vi "fucking cubes.vi"() -> ()   [LabVIEW 2010]
uses:
  <vilib>/Analysis/Matrix/Datatypes/RealMatrix.ctl
  <vilib>/picture/3D Picture Control/NI_3D Picture Control.lvlib
  <vilib>/Analysis/Matrix/NI_Matrix.lvlib
panel:
  out "Supercell Structure":T1={"Structure Name"="A3B3_twin", "Lattice vector a"=[4.67354, 0.0, 0.0], "Lattice vector b"=[0.0, 8.0948, 0.0], "Lattice vector c"=[0.0, 0.0, 22.8956], "Atoms Array"=[{"Atom Name"="Cd", "Positions (Direct)"=[[0.0, 0.3333160110632741, 0.0416917449166463], [0.5000009999999975, 0.8333170110632716, 0.0416917449166463], [0.5000009999999975, 0.1666621408709168, 0.208337818520255], [0.0, 0.6666631408709214, 0.208337818520255], [0.0, 8.4662249422e-06, 0.3749383421346864], [0.5000009999999975, 0.5000094662249397, 0.3749383421346864], [0.0, -8.4662249422e-06, 0.8749383421346864], [0.5000009999999975, 0.4999925337750553, 0.8749383421346864], [0.0, 0.3333388591290807, 0.7083368185202576], [0.5000009999999975, 0.8333398591290782, 0.7083368185202576], [0.5000009999999975, 0.1666849889367233, 0.5416917449166463], [0.0, 0.6666859889367279, 0.5416917449166463]], "Positions (Cartesian)"=[[0.0, 2.6981264463549905, 0.9545575149135672], [2.3367746735399884, 6.745534541154971, 0.9545575149135672], [2.3367746735399884, 1.3490966979218972, 4.770019357712351], [0.0, 5.396504792721934, 4.770019357712351], [0.0, 6.853239766212056e-05, 8.584438306178926], [2.3367746735399884, 4.047476627197642, 8.584438306178926], [0.0, -6.853239766212056e-05, 20.032238306178925], [2.3367746735399884, 4.047339562402318, 20.032238306178925], [0.0, 2.698311396878082, 16.217796462112414], [2.3367746735399884, 6.745719491678061, 16.217796462112414], [2.3367746735399884, 1.3492816484449877, 12.402357514913568], [0.0, 5.396689743245025, 12.402357514913568]]}, {"Atom Name"="Te", "Positions (Direct)"=[[0.0, -2.2822775934e-06, 0.0001327438415307], [0.5000009999999975, 0.499998717722404, 0.0001327438415307], [0.0, 0.3333991470731503, 0.166602258546053], [0.5000009999999975, 0.8334001470731478, 0.166602258546053], [0.5000009999999975, 0.1666248769120535, 0.3332990920408234], [0.0, 0.6666258769120581, 0.3332990920408234], [0.0, 0.333376123087944, 0.8332980920408259], [0.5000009999999975, 0.8333771230879414, 0.8332980920408259], [0.5000009999999975, 0.1666018529268472, 0.6666022585460529], [0.0, 0.6666028529268517, 0.6666022585460529], [0.0, 2.2822775934e-06, 0.5001327438415307], [0.5000009999999975, 0.5000032822775909, 0.5001327438415307]], "Positions (Cartesian)"=[[0.0, -1.8474580663054318e-05, 0.003039249898150295], [2.3367746735399884, 4.047389620219316, 0.003039249898150295], [0.0, 2.698799415727737, 3.814458670767012], [2.3367746735399884, 6.746207510527716, 3.814458670767012], [2.3367746735399884, 1.3487950536276905, 7.631082691729877], [0.0, 5.396203148427728, 7.631082691729877], [0.0, 2.698613041172289, 19.078859796129937], [2.3367746735399884, 6.746021135972268, 19.078859796129937], [2.3367746735399884, 1.3486086790722427, 15.262258670767011], [0.0, 5.396016773872279, 15.262258670767011], [0.0, 1.8474580663054318e-05, 11.450839249898152], [2.3367746735399884, 4.047426569380643, 11.450839249898152]]}], "# of atoms"=24}
  out "Grain 1 Object":refnum<vi>
  out "Grain 1 Render":refnum<vi>(3d-picture)
  in  "Conventional Unit Cell":T1={"Structure Name"="CdTe", "Lattice vector a"=[6.615785553057252, 0.0, 0.0], "Lattice vector b"=[0.0, 6.615785553057252, 0.0], "Lattice vector c"=[0.0, 0.0, 6.615785553057252], "Atoms Array"=[{"Atom Name"="Cd", "Positions (Direct)"=[[0.0, 0.0, 0.0], [0.0, 0.5, 0.5], [0.5, 0.0, 0.5], [0.5, 0.5, 0.0]], "Positions (Cartesian)"=[[0.0, 0.0, 0.0], [0.0, 3.307892776528626, 3.307892776528626], [3.307892776528626, 0.0, 3.307892776528626], [3.307892776528626, 3.307892776528626, 0.0]]}, {"Atom Name"="Te", "Positions (Direct)"=[[0.25, 0.25, 0.25], [0.75, 0.75, 0.25], [0.75, 0.25, 0.75], [0.25, 0.75, 0.75]], "Positions (Cartesian)"=[[1.653946388264313, 1.653946388264313, 1.653946388264313], [4.96183916479294, 4.96183916479294, 1.653946388264313], [4.96183916479294, 1.653946388264313, 4.96183916479294], [1.653946388264313, 4.96183916479294, 4.96183916479294]]}], "# of atoms"=8}
  in  "Slide":i32(slide) scale=0.0..4.0
  out "Array":cluster{"Rotation Matrix":T2}[](array[cluster])
  in  "System Array":cluster{"Axis":dbl[], "Angle":dbl}[](array[cluster])
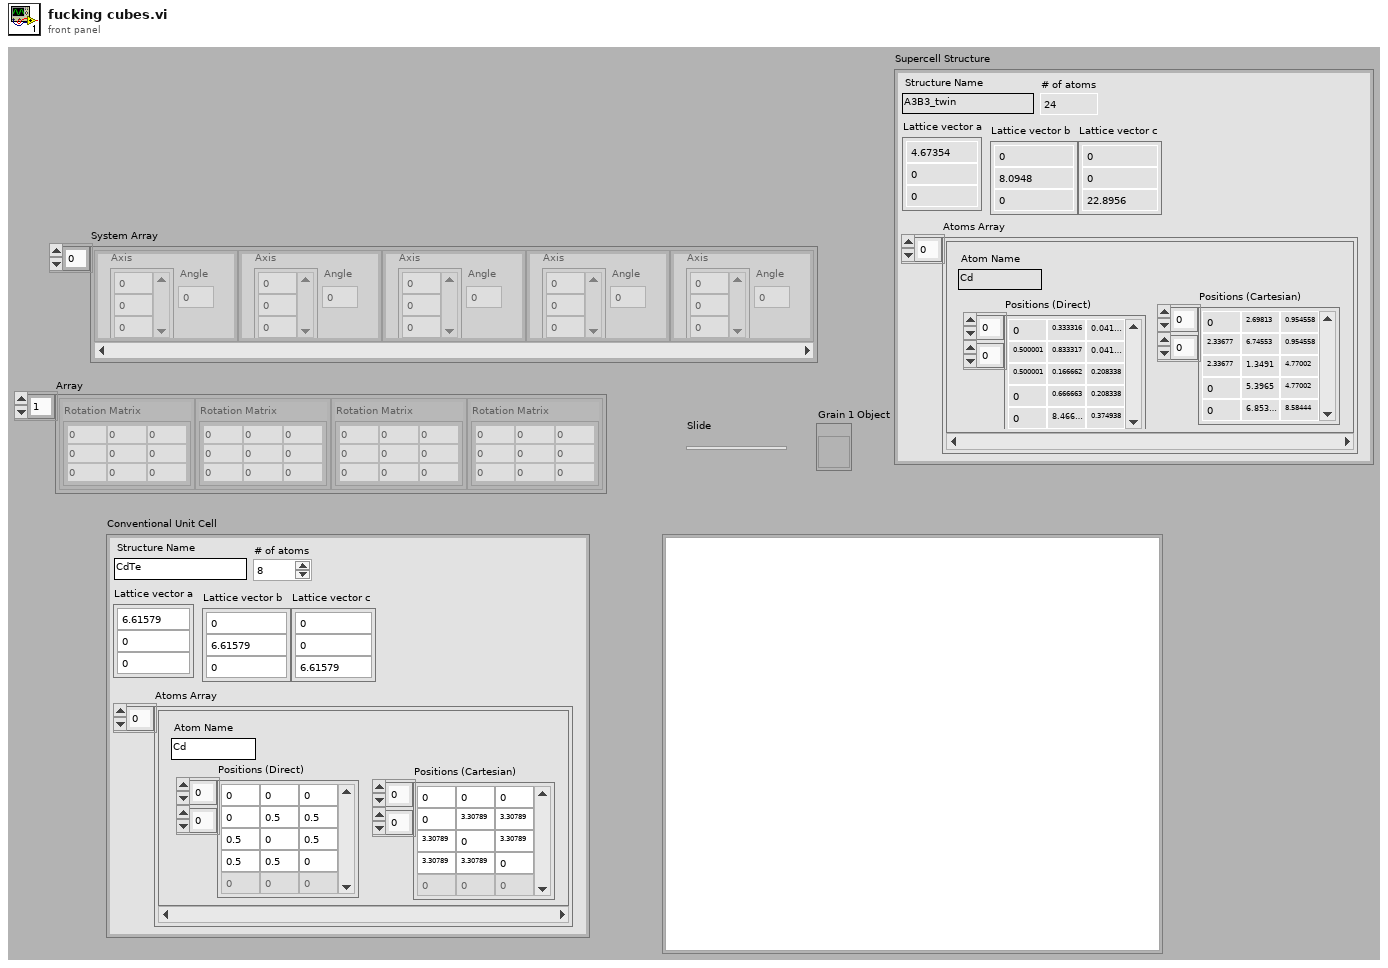
[diagram p1: front panel]
types:
  T1 = cluster{"Structure Name":string, "Lattice vector a":dbl[], "Lattice vector b":dbl[], "Lattice vector c":dbl[], "Atoms Array":cluster{"Atom Name":string, "Positions (Direct)":dbl[][], "Positions (Cartesian)":dbl[][]}[], "# of atoms":i32}
  T2 = typedef "NI_Matrix.lvlib/RealMatrix.ctl" = dbl[][]
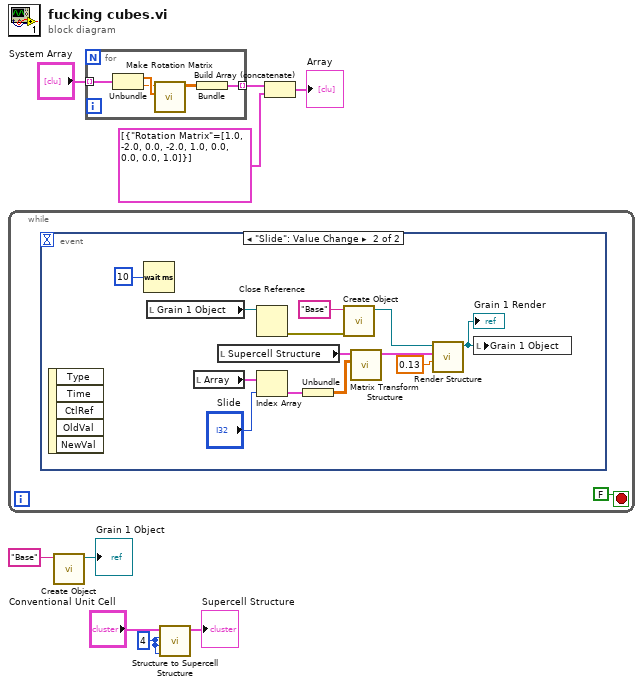
[diagram p0: block diagram]
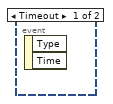
[diagram p2: hidden frame]
diagram:
  w2 = i16 4 ("a lattice factor")
  n1 = while {
    stop <- FALSE stop-if-true
    n2 = event shown="[1] \"Slide\": Value Change" {
      selector: _ -> [_ _]
      dyn-events: _ -> [_ _]
      timeout: _ -> [_ _]
      event Timeout {
        n3 = event-data() -> ()  [unwired: 1 in, 2 out]
      }
      event "Slide": Value Change {
        n4 = event-data() -> ()  [unwired: 1 in, 5 out]
        n5 = Wait (ms)(milliseconds to wait=u32 10) -> ()  [unwired: 1 out]
        n6 = local read "Grain 1 Object"() -> (w16:refnum<vi>)
        n7 = local read "Array"() -> (w20:cluster{"Rotation Matrix":T2}[])
        n8 = local read "Supercell Structure"() -> (w11:T1)
        n9 = Close Reference(reference=w16) -> (error out=w17:errorcluster)  [unwired: 1 in]
        n10 = Index Array(array=w20, index="Slide") -> (element=w22:cluster{"Rotation Matrix":T2})
        n11 = Unbundle(w22) -> ("Rotation Matrix"=w23:T2)
        n12 = call <vilib>:"Create Object.vi"("error in (no error)"=w17, "Name"="Base") -> ("Scene:New Object"=w15:refnum<vi>)  [unwired: 9 out]
        n13 = call "Matrix Transform Structure.vi"("Matrix Transform"=w23, "Original Structure"=w11) -> ("After Transform"=w13:T1)  [unwired: 9 in]
        n14 = call "Render Structure.vi"("Scale"=0.13, "Atomic Structure"=w13, "Base Object"=w15) -> ("Object with atoms"=w18:refnum<vi>)  [unwired: 8 in]
        "Grain 1 Render" <- w18
        n15 = local write "Grain 1 Object"(w18) -> ()
      }
    }
  }
  n16 = call <vilib>:"Create Object.vi"("Name"="Base") -> ("Scene:New Object"=→"Grain 1 Object":refnum<vi>)  [unwired: 1 in, 9 out]
  n17 = for {
    tunnel: "System Array" -> [w28] mode=indexing
    tunnel: [w24] -> w6 mode=indexing
    n18 = Unbundle(w28) -> ("Axis"=w27:dbl[], "Angle"=w26:dbl)
    n19 = call "Make Rotation Matrix.vi"("Rotation Axis"=w27, "Rotation Angle (Degree)"=w26) -> ("Rotation Matrix"=w25:T2)  [unwired: 9 in]
    n20 = Bundle("Rotation Matrix"=w25) -> (w24:cluster{"Rotation Matrix":T2})  [unwired: 1 in]
  }
  n21 = call "Structure to Supercell Structure.vi"("c lattice factor"=w2, "b lattice factor"=w2, "a lattice factor"=w2, "Input Structure"="Conventional Unit Cell") -> ("Supercell Structure"=→"Supercell Structure":T1)  [unwired: 7 in]
  n22 = Build Array (concatenate)(w6, cluster{"Rotation Matrix":T2}[] [{"Rotation Matrix"=[[1.0, -2.0, 0.0], [-2.0, 1.0, 0.0], [0.0, 0.0, 1.0]]}] ("element")) -> (→"Array":cluster{"Rotation Matrix":T2}[])
